vi "组合框学习.vi"() -> ()   [LabVIEW 2018]
panel:
  out "密码显示":string
  out "正常显示":string
  in  "组合框":string(combo)
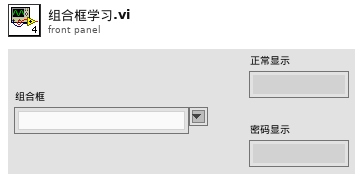
[diagram p1: front panel]
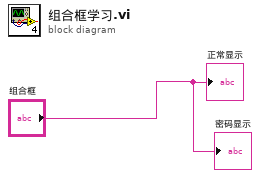
[diagram p0: block diagram]
diagram:
  "正常显示" <- "组合框"
  "密码显示" <- "组合框"
